vi "Teleop.vi"(10 "Match Info":T2={"Autonomous Elapsed Seconds"=0.0, "TeleOp Elapsed Seconds"=0.0, "Disabled Elapsed Seconds"=0.0, "Visited Autonomous"=FALSE, "Visited TeleOp"=FALSE, "Visited Disabled"=FALSE, "Autonomous Settings"={"Autonomous Style"=enum."Independent", "VI Refnum"=refnum}}, 11 "Call Context":T3) -> ()   [LabVIEW 2015]
doc: "This VI is called for each TeleOp packet received from the DS where the robot is not disabled. It is often used to read from the joysticks and update I/O or to update setpoints for timed control loops. It should complete and return within 20 milliseconds or it may miss DS packets."
uses:
  <vilib>/Rock Robotics/WPI/DriverStation/WPI_DriverStationDerivedRobotMode.ctl
  <vilib>/Rock Robotics/WPI/DriverStation/WPI_DriverStationMatch Info.ctl
  <vilib>/Rock Robotics/WPI/Utilities/WPI_GetSetVariantRefNum.vi
  <vilib>/addons/control/pid/pid.llb/PID (DBL).vi
  Robot Global Data.vi
  <vilib>/addons/control/pid/NI_PID_pid.lvlib
panel:
  in  "PID Gains Right":T1={"proportional gain (Kc)"=1.0, "integral time (Ti, min)"=0.01, "derivative time (Td, min)"=0.0} {"derivative time (Td, min)" format="%.3f"; "integral time (Ti, min)" format="%.3f"; "proportional gain (Kc)" format="%.3f"}
  out "Left Drive":dbl[](graph)
  out "Right Drive":dbl[](graph)
  in  "PID Gains Left":T1={"proportional gain (Kc)"=1.0, "integral time (Ti, min)"=0.01, "derivative time (Td, min)"=0.0} {"derivative time (Td, min)" format="%.3f"; "integral time (Ti, min)" format="%.3f"; "proportional gain (Kc)" format="%.3f"}
  in  "Range":cluster{"output high":dbl, "output low":dbl}={"output high"=100.0, "output low"=-100.0} {"output low" format="%.2f"; "output high" format="%.2f"}
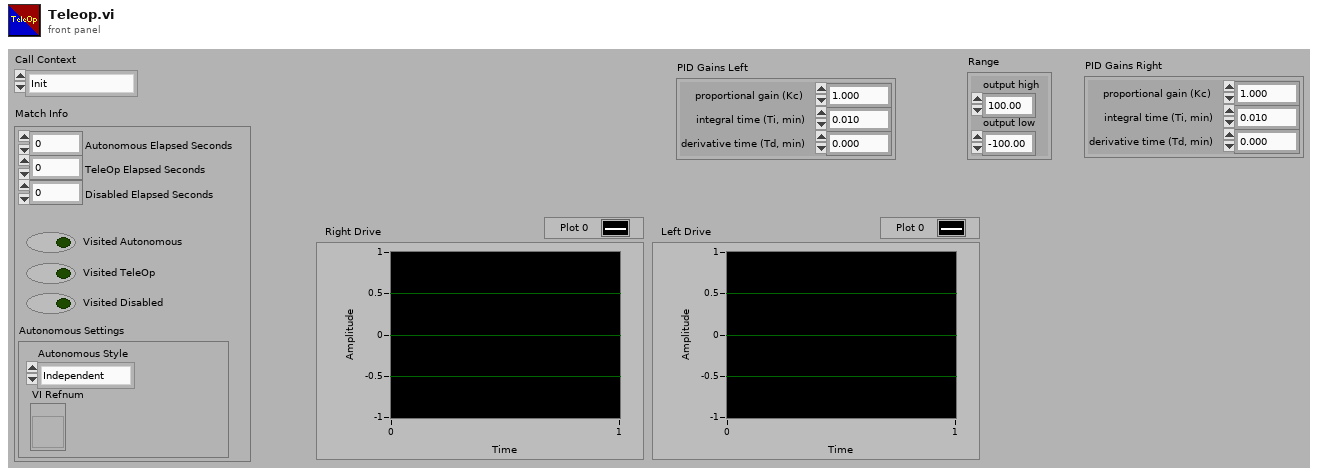
[diagram p1: front panel]
types:
  T1 = cluster{"proportional gain (Kc)":dbl, "integral time (Ti, min)":dbl, "derivative time (Td, min)":dbl}
  T2 = typedef "WPI_DriverStationMatch Info.ctl" = cluster{"Autonomous Elapsed Seconds":dbl, "TeleOp Elapsed Seconds":dbl, "Disabled Elapsed Seconds":dbl, "Visited Autonomous":bool, "Visited TeleOp":bool, "Visited Disabled":bool, "Autonomous Settings":cluster{"Autonomous Style":enum16{"Iterative", "Independent"}, "VI Refnum":refnum<vi>}}
  T3 = typedef "WPI_DriverStationDerivedRobotMode.ctl" = enum16{"Init", "Execute", "Stop"}
  T4 = typedef "WPI_JoystickDevRef.ctl" = cluster{"Device":T5}
  T5 = typedef "WPI_JoystickDeviceEnum.ctl" = enum16{"USB 0", "USB 1", "USB 2", "USB 3", "USB 4", "USB 5"}
  T6 = cluster{"Axes[0]":dbl, "Axes[1]":dbl, "Axes[2]":dbl, "Axes[3]":dbl, "Axes[4]":dbl, "Axes[5]":dbl, "Axes[6]":dbl, "Axes[7]":dbl, "Axes[8]":dbl}
  T7 = typedef "WPI_EncoderDevRef.ctl" = cluster{"DevStatus":errorcluster, "EncoderIndex":T8, "CounterIndex":T9, "DistancePerCount":dbl, "Decoding Type":T10}
  T8 = typedef "FPGA_EncoderIdx.ctl" = enum8{"Enc 0", "Enc 1", "Enc 2", "Enc 3", "Enc 4", "Enc 5", "Enc 6", "Enc 7", "Invalid"}
  T9 = typedef "FPGA_CounterCtrSystemIndex.ctl" = enum8{"Ctr 0", "Ctr 1", "Ctr 2", "Ctr 3", "Ctr 4", "Ctr 5", "Ctr 6", "Ctr 7", "Invalid"}
  T10 = typedef "WPI_EncoderType.ctl" = enum16{"1x", "2x", "4x"}
  T11 = typedef "WPI_RobotDriveDevRef.ctl" = cluster{"DevStatus":errorcluster, "Motors[]":T12[], "Square Inputs":bool, "Max Output":dbl}
  T12 = typedef "WPI_MotorControlDeviceRef.ctl" = cluster{"DeviceStatus":errorcluster, "Type":T13, "PWM":cluster{"PWM Channel":T14, "DeadBand":T15}, "CAN":cluster{"Device Number":u8, "Control Mode":T16, "Semaphore":T17, "Max Vout":dbl, "TalonSRX Control Mode":T18}, "Invert":bool}
  T13 = typedef "WPI_MotorControlType.ctl" = enum16{"PWM", "CAN", "CANTalonSRX"}
  T14 = typedef "FPGA_DIOPWMChannel.ctl" = enum8{"PWM 0", "PWM 1", "PWM 2", "PWM 3", "PWM 4", "PWM 5", "PWM 6", "PWM 7", "PWM 8", "PWM 9", "PWM MXP 0", "PWM MXP 1", "PWM MXP 2", "PWM MXP 3", "PWM MXP 4", "PWM MXP 5", "PWM MXP 6", "PWM MXP 7", "PWM MXP 8", "PWM MXP 9", "Invalid"}
  T15 = typedef "WPI_PWMDeadband.ctl" = cluster{"Name":string, "maxPositivePwm":i32, "minPositivePwm":i32, "centerPwm":i32, "maxNegativePwm":i32, "minNegativePwm":i32, "angularRange":u16}
  T16 = typedef "WPI_CANJaguar_ControlMode.ctl" = enum8{"Percent VBus", "Current", "Speed", "Position", "Voltage"}
  T17 = typedef "Semaphore RefNum" = refnum<k1>
  T18 = typedef "WPI_CANTalonSRX_APIControlMode.ctl" = enum8{"Percent VBus", "Speed", "Position", "Slave", "Unchanged / Invalid", "Voltage Compensation", "Current", "Motion Profile"}
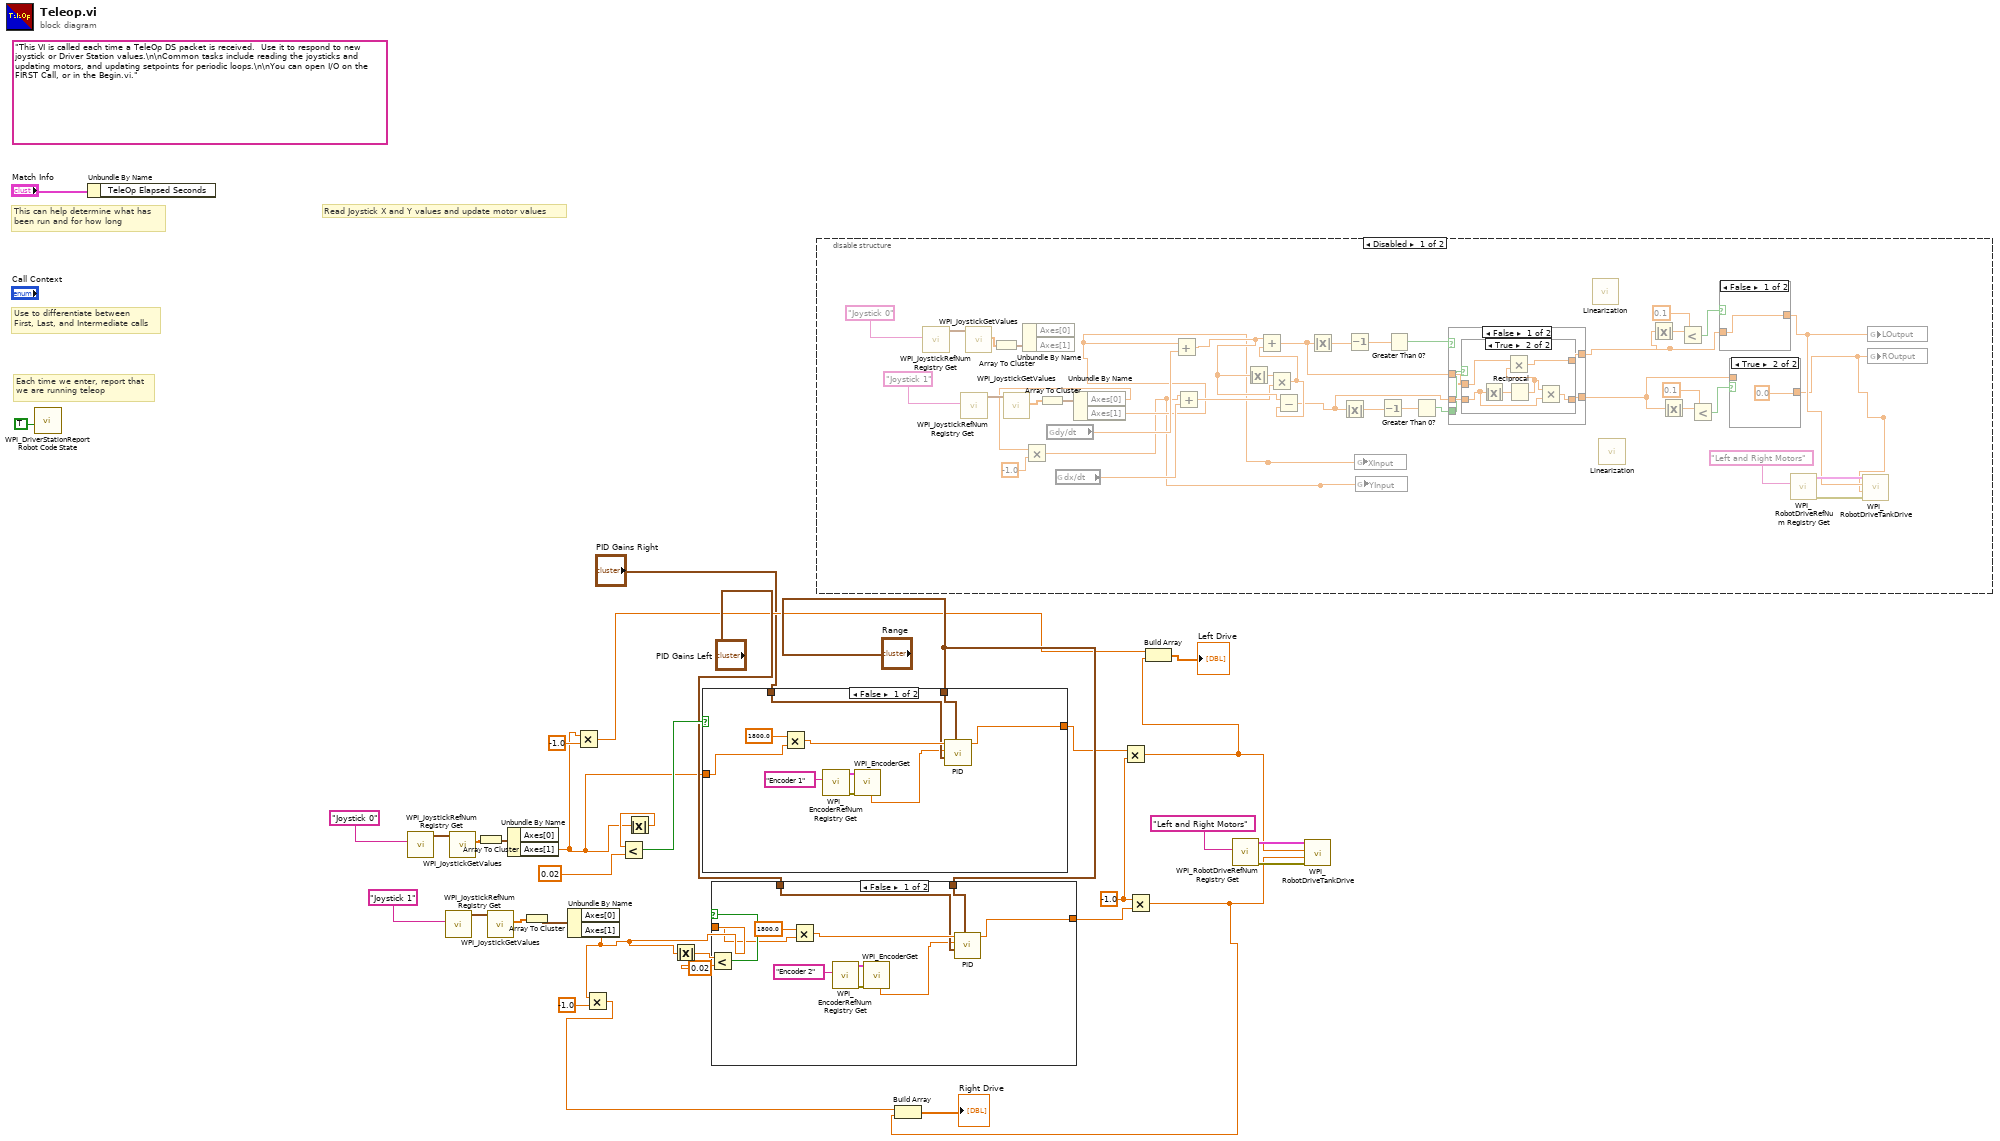
[diagram p0: block diagram]
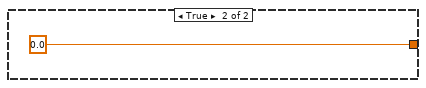
[diagram p2: hidden frame]
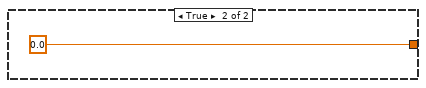
[diagram p3: hidden frame]
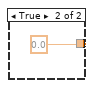
[diagram p5: hidden frame]
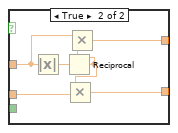
[diagram p7: hidden frame]
diagram:
  w14 = -1.0 ("x")
  (unwired) "This VI is called each time a TeleOp DS packet is received.  Use it to respond to new joystick or Driver Station values.\n\nCommon tasks include reading the joysticks and updating motors, and updating setpoints for periodic loops.\n\nYou can open I/O on the FIRST Call, or in the Begin.vi."
  # "Each time we enter, report that\nwe are running teleop"
  # "Use to differentiate between\nFirst, Last, and Intermediate calls"
  # "This can help determine what has\nbeen run and for how long"
  # "Read Joystick X and Y values and update motor values"
  n1 = call <vilib>:"WPI_DriverStationReport Robot Code State.vi"("TeleOp"=TRUE ("Autonomous")) -> ()  [unwired: 10 in, 1 out]
  n2 = Unbundle By Name("Match Info") -> ()  [unwired: 1 out]
  n3 = call <vilib>:"WPI_JoystickRefNum Registry Get.vi"("refnum name"="Joystick 0") -> ("JoystickDevRef"=w32:T4)  [unwired: 1 in, 9 out]
  n4 = call <vilib>:"WPI_JoystickRefNum Registry Get.vi"("refnum name"="Joystick 1") -> ("JoystickDevRef"=w30:T4)  [unwired: 1 in, 9 out]
  n5 = call <vilib>:"WPI_JoystickGetValues.vi"("JoystickDevRef"=w32) -> ("Axes"=w27:dbl[])  [unwired: 6 in, 4 out]
  n6 = Array To Cluster(array=w27) -> (cluster=w26:T6)
  n7 = call <vilib>:"WPI_JoystickGetValues.vi"("JoystickDevRef"=w30) -> ("Axes"=w29:dbl[])  [unwired: 6 in, 4 out]
  n8 = Unbundle By Name(w26) -> ("Axes[1]"=w1:dbl)  [unwired: 1 out]
  n9 = Array To Cluster(array=w29) -> (cluster=w28:T6)
  n10 = Unbundle By Name(w28) -> ("Axes[1]"=w4:dbl)  [unwired: 1 out]
  n11 = Multiply(x=w1, y=-1.0) -> (x*y=w7:dbl)
  n12 = Multiply(x=w4, y=-1.0) -> (x*y=w11:dbl)
  n13 = Absolute Value(x=w1) -> (abs(x)=w2:dbl)
  n14 = Less?(x=w2, y=0.02) -> (x < y?=w24:bool)
  n15 = Absolute Value(x=w4) -> (abs(x)=w3:dbl)
  n16 = case shown="False" w24 {
    tunnel: [w40 0.0] -> w15
    tunnel: "Range" -> [w39 _]
    tunnel: "PID Gains Right" -> [w38 _]
    tunnel: w1 -> [w36 _]
    frame False {
      n17 = Multiply(x=1800.0, y=w36) -> (x*y=w42:dbl)
      n18 = call <vilib>:"WPI_EncoderRefNum Registry Get.vi"("refnum name"="Encoder 1") -> ("error out"=w43:errorcluster, "EncoderDevRef"=w44:T7)  [unwired: 9 in]
      n19 = call <vilib>:"WPI_EncoderGet.vi"("error in (no error)"=w43, "EncoderDevRef"=w44) -> ("Rate"=w37:dbl)  [unwired: 4 in, 5 out]
      n20 = call-poly <vilib>:"PID.vi"("output range"=w39, "PID gains"=w38, "process variable"=w37, "setpoint"=w42) -> ("output"=w40:dbl)  [unwired: 6 in, 1 out]
    }
    frame True {
    }
  }
  n21 = Less?(x=w3, y=0.02) -> (x < y?=w19:bool)
  n22 = case shown="False" w19 {
    tunnel: w4 -> [w50 _]
    tunnel: [w51 0.0] -> w16
    tunnel: "Range" -> [w49 _]
    tunnel: "PID Gains Left" -> [w48 _]
    frame False {
      n23 = Multiply(x=1800.0, y=w50) -> (x*y=w53:dbl)
      n24 = call <vilib>:"WPI_EncoderRefNum Registry Get.vi"("refnum name"="Encoder 2") -> ("error out"=w54:errorcluster, "EncoderDevRef"=w55:T7)  [unwired: 9 in]
      n25 = call <vilib>:"WPI_EncoderGet.vi"("error in (no error)"=w54, "EncoderDevRef"=w55) -> ("Rate"=w47:dbl)  [unwired: 4 in, 5 out]
      n26 = call-poly <vilib>:"PID.vi"("output range"=w49, "PID gains"=w48, "process variable"=w47, "setpoint"=w53) -> ("output"=w51:dbl)  [unwired: 6 in, 1 out]
    }
    frame True {
    }
  }
  n27 = disable-structure shown="Disabled" {
    frame Disabled {
      n28 = call <vilib>:"WPI_JoystickRefNum Registry Get.vi"("refnum name"="Joystick 0") -> ("JoystickDevRef"=w94:T4)  [unwired: 1 in, 9 out]
      n29 = call <vilib>:"WPI_JoystickRefNum Registry Get.vi"("refnum name"="Joystick 1") -> ("JoystickDevRef"=w92:T4)  [unwired: 1 in, 9 out]
      n30 = call <vilib>:"WPI_JoystickGetValues.vi"("JoystickDevRef"=w94) -> ("Axes"=w89:dbl[])  [unwired: 6 in, 4 out]
      n31 = Array To Cluster(array=w89) -> (cluster=w88:T6)
      n32 = call <vilib>:"WPI_JoystickGetValues.vi"("JoystickDevRef"=w92) -> ("Axes"=w91:dbl[])  [unwired: 6 in, 4 out]
      n33 = Unbundle By Name(w88) -> ()  [unwired: 2 out]
      n34 = Array To Cluster(array=w91) -> (cluster=w90:T6)
      n35 = global read "Robot Global Data.vi" "dy/dt"() -> (w77:dbl)
      n36 = global read "Robot Global Data.vi" "dx/dt"() -> (w75:dbl)
      n37 = Unbundle By Name(w90) -> ("Axes[0]"=w59:dbl, "Axes[1]"=w61:dbl)
      n38 = Multiply(x=w59, y=-1.0) -> (x*y=w58:dbl)
      n39 = Add(x=w61, y=w77) -> (x+y=w76:dbl)
      n40 = Add(x=w58, y=w75) -> (x+y=w74:dbl)
      n41 = Absolute Value(x=w76) -> (abs(x)=w87:dbl)
      n42 = Multiply(x=w87, y=w74) -> (x*y=w86:dbl)
      n43 = Add(x=w76, y=w86) -> (x+y=w81:dbl)
      n44 = Subtract(x=w76, y=w86) -> (x-y=w79:dbl)
      n45 = Absolute Value(x=w81) -> (abs(x)=w85:dbl)
      n46 = Absolute Value(x=w79) -> (abs(x)=w84:dbl)
      n47 = Decrement(x=w85) -> (x-1=w80:dbl)
      n48 = global write "Robot Global Data.vi" "XInput"(w61) -> ()
      n49 = global write "Robot Global Data.vi" "YInput"(w58) -> ()
      n50 = Decrement(x=w84) -> (x-1=w83:dbl)
      n51 = Greater Than 0?(x=w80) -> (x > 0?=w82:bool)
      n52 = Greater Than 0?(x=w83) -> (x > 0?=w78:bool)
      n53 = case shown="False" w82 {
        tunnel: w81 -> [w105 w116]
        tunnel: w79 -> [w104 w118]
        tunnel: [w101 w115] -> w63
        tunnel: [w102 w114] -> w62
        tunnel: w78 -> [w103 _]
        frame False {
          n54 = case shown="True" w103 {
            tunnel: w105 -> [w107 w112]
            tunnel: w104 -> [w106 w109]
            tunnel: [w107 w111] -> w101
            tunnel: [w106 w108] -> w102
            frame False {
            }
            frame True {
              n55 = Absolute Value(x=w109) -> (abs(x)=w113:dbl)
              n56 = Reciprocal(x=w113) -> (1/x=w110:dbl)
              n57 = Multiply(x=w112, y=w110) -> (x*y=w111:dbl)
              n58 = Multiply(x=w110, y=w109) -> (x*y=w108:dbl)
            }
          }
        }
        frame True {
          n59 = Absolute Value(x=w116) -> (abs(x)=w119:dbl)
          n60 = Reciprocal(x=w119) -> (1/x=w117:dbl)
          n61 = Multiply(x=w117, y=w118) -> (x*y=w114:dbl)
          n62 = Multiply(x=w116, y=w117) -> (x*y=w115:dbl)
        }
      }
      n63 = call "Linearization.vi"() -> ()  [unwired: 1 in, 1 out]
      n64 = call "Linearization.vi"() -> ()  [unwired: 1 in, 1 out]
      n65 = Absolute Value(x=w63) -> (abs(x)=w73:dbl)
      n66 = Absolute Value(x=w62) -> (abs(x)=w70:dbl)
      n67 = Less?(x=w73, y=0.1) -> (x < y?=w71:bool)
      n68 = Less?(x=w70, y=0.1) -> (x < y?=w68:bool)
      n69 = case shown="False" w71 {
        tunnel: [w99 0.0] -> w65
        tunnel: w63 -> [w99 _]
        frame False {
        }
        frame True {
        }
      }
      n70 = case shown="True" w68 {
        tunnel: [w97 0.0] -> w64
        tunnel: w62 -> [w97 _]
        frame False {
        }
        frame True {
        }
      }
      n71 = call <vilib>:"WPI_RobotDriveRefNum Registry Get.vi"("refnum name"="Left and Right Motors") -> ("error out"=w66:errorcluster, "RobotDriveDevRef"=w67:T11)  [unwired: 1 in, 8 out]
      n72 = call <vilib>:"WPI_RobotDriveTankDrive.vi"("error in (no error)"=w66, "Right axis value"=w64, "Left axis value"=w65, "RobotDriveDevRef"=w67) -> ()  [unwired: 5 in, 3 out]
      n73 = global write "Robot Global Data.vi" "LOutput"(w65) -> ()
      n74 = global write "Robot Global Data.vi" "ROutput"(w64) -> ()
    }
    frame Enabled {
    }
  }
  n75 = Multiply(x=w15, y=w14) -> (x*y=w6:dbl)
  n76 = Multiply(x=w14, y=w16) -> (x*y=w10:dbl)
  n77 = Build Array(w11, w10) -> (→"Right Drive":dbl[])
  n78 = Build Array(w7, w6) -> (→"Left Drive":dbl[])
  n79 = call <vilib>:"WPI_RobotDriveRefNum Registry Get.vi"("refnum name"="Left and Right Motors") -> ("error out"=w20:errorcluster, "RobotDriveDevRef"=w21:T11)  [unwired: 1 in, 8 out]
  n80 = call <vilib>:"WPI_RobotDriveTankDrive.vi"("error in (no error)"=w20, "Right axis value"=w10, "Left axis value"=w6, "RobotDriveDevRef"=w21) -> ()  [unwired: 5 in, 3 out]
